vi "Add Rows.vi"(8 "error in (no error)":errorcluster, 10 "Cells":T2(array[cluster]), 11 "DataGridView in":refnum<class "DataGridView.lvclass">) -> (0 "error out":errorcluster, 3 "DataGridView out":refnum<class "DataGridView.lvclass">)   [LabVIEW 2013, in "DataGrid.lvlib" / "DataGridView.lvclass"]
doc: "This method allows you to add any rows of any time, regardless of the data column setup."
uses:
  DataGridView.lvclass
  GridColumn/ColumnType.ctl
  DataGridView.lvclass/DataGridView.ctl
  System.Windows.Forms
  DataTable/DataTable.lvclass
  GridColumn/GridColumn.lvclass
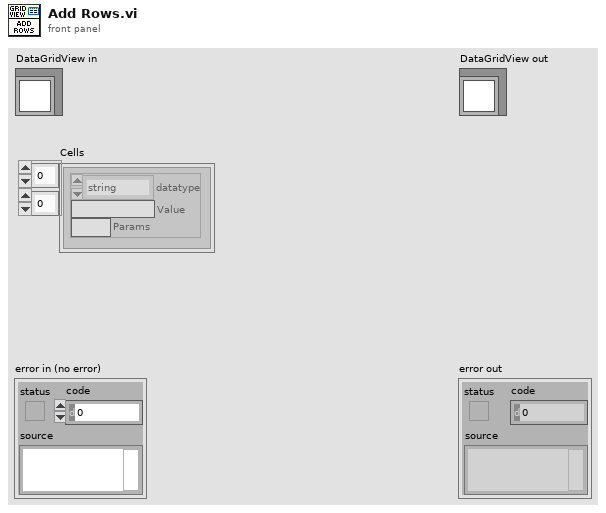
[diagram p1: front panel]
types:
  T1 = typedef "DataGrid.lvlib/GridColumn.lvclass/ColumnType.ctl" = enum16{"string", "image", "check", "numeric", "timestamp", "button", "combo", "link"}
  T2 = cluster{"datatype":T1, "Value":string, "Params":string}[][]
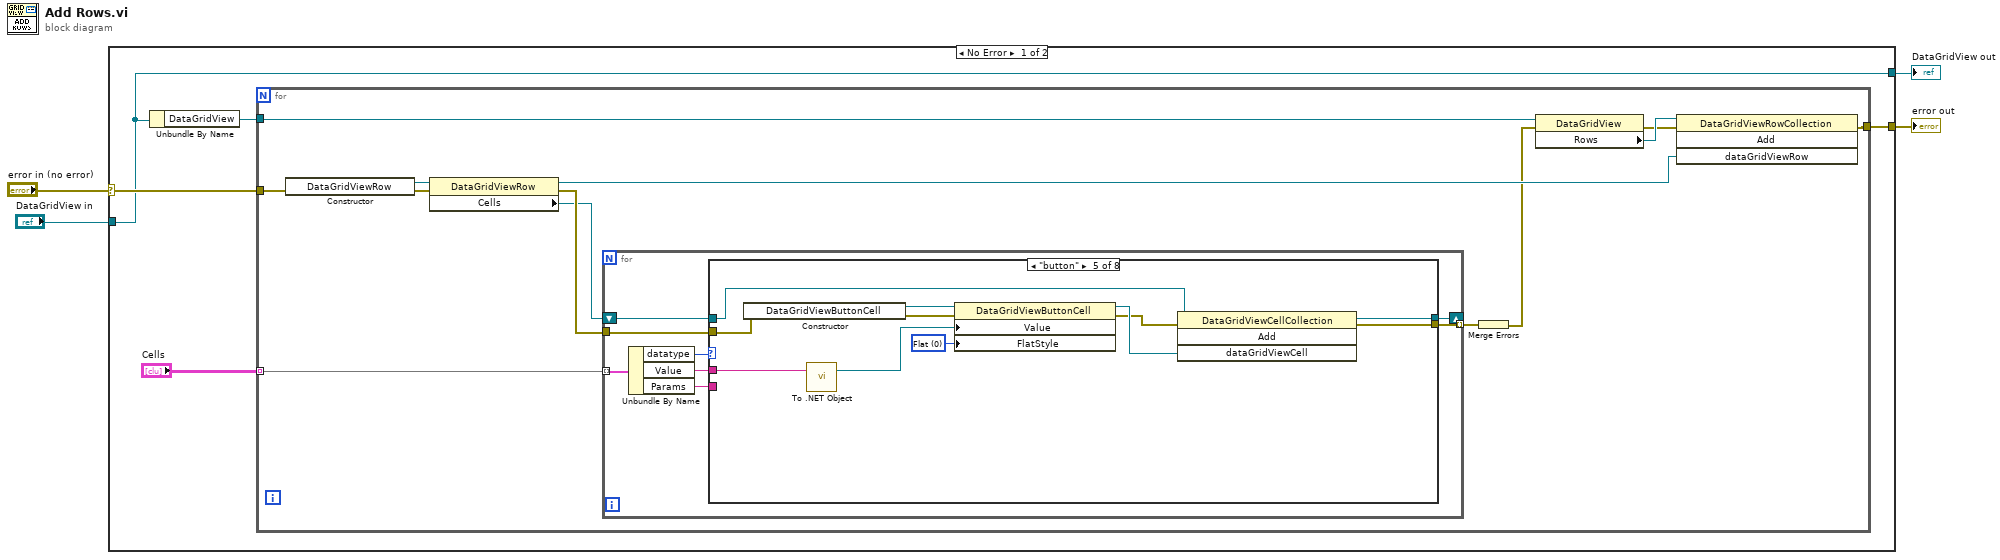
[diagram p0: block diagram]
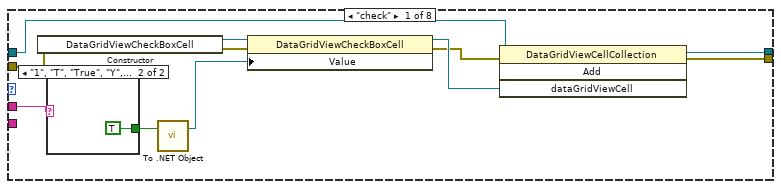
[diagram p2: hidden frame]
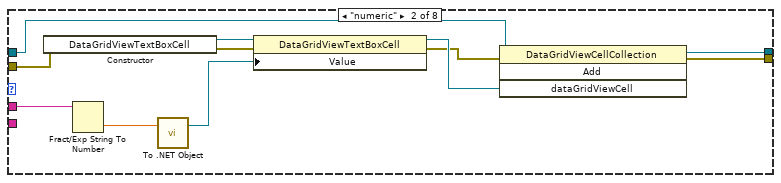
[diagram p4: hidden frame]
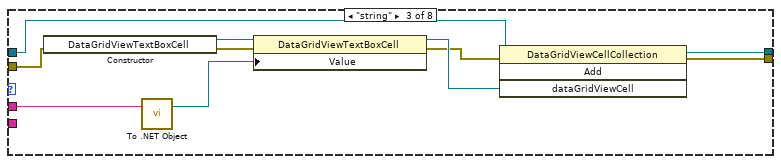
[diagram p5: hidden frame]
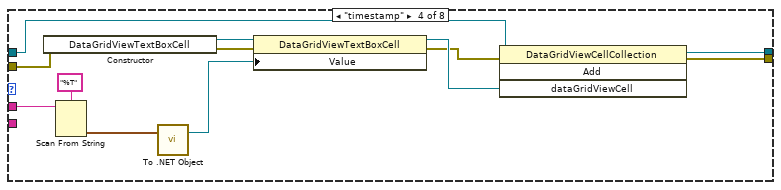
[diagram p6: hidden frame]
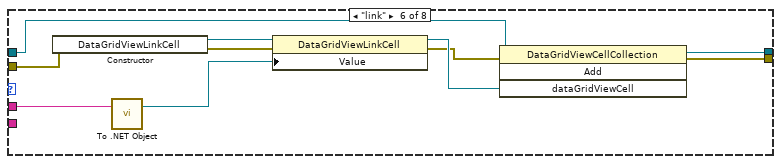
[diagram p7: hidden frame]
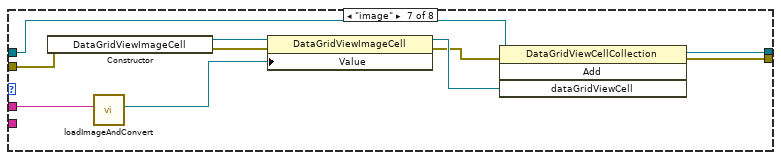
[diagram p8: hidden frame]
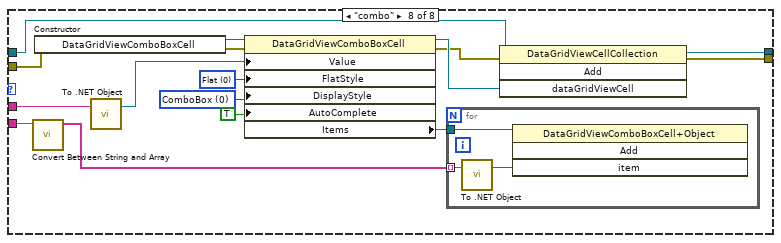
[diagram p9: hidden frame]
diagram:
  n1 = case shown="No Error" "error in (no error)" {
    selector: "error in (no error)" -> [w7 w127]
    tunnel: [w9 w127] -> w3
    tunnel: [w5 w126] -> w1
    tunnel: "DataGridView in" -> [w5 w126]
    frame No Error {
      n2 = Unbundle By Name(w5) -> ("DataGridView"=w8:refnum<k24>)
      n3 = for {
        tunnel: [w22] -> w9
        tunnel: w8 -> [w21]
        tunnel: w7 -> [w17]
        tunnel: "Cells" -> [w10] mode=indexing
        n4 = constructor class="DataGridViewRow"(error in=w17) -> (reference out=w15:refnum<k24>, error out=w16:errorcluster)  [unwired: 2 in, 1 out]
        n5 = property class="DataGridViewRow"(reference=w15, error in=w16) -> (reference out=w14:refnum<k24>, error out=w12:errorcluster, "Cells"=w11:refnum<k24>)
        n6 = for {
          tunnel: w10 -> [w30] mode=indexing
          shift-right: [w26] -> _
          shift-left: w11 -> [w25]
          tunnel: w12 -> [w24]
          tunnel: [w23] -> w19 mode=indexing
          n7 = Unbundle By Name(w30) -> ("datatype"=w29:T1, "Value"=w28:string, "Params"=w27:string)
          n8 = case shown="\"button\"" w29 {
            tunnel: w28 -> [w40 w47 w57 w68 w79 w90 w101 w109]
            tunnel: w27 -> [_ _ _ _ _ _ _ w116]
            tunnel: [w37 w51 w61 w73 w84 w94 w104 w120] -> w26
            tunnel: w25 -> [w35 w49 w59 w71 w82 w92 w102 w118]
            tunnel: w24 -> [w33 w43 w56 w66 w76 w89 w99 w111]
            tunnel: [w31 w45 w54 w65 w77 w87 w98 w113] -> w23
            frame "check" {
              n9 = constructor class="DataGridViewCheckBoxCell"(error in=w33) -> (reference out=w38:refnum<k24>, error out=w39:errorcluster)  [unwired: 2 in, 1 out]
              n10 = case shown="\"1\", \"T\", \"True\", \"Y\", \"Yes\"" w40 {
                tunnel: [_ TRUE] -> w41
                frame Default {
                }
                frame "1", "T", "True", "Y", "Yes" {
                }
              }
              n11 = call <vilib>:"To .NET Object.vi"("anything"=w41) -> (".NET object"=w34:refnum<k24>)  [unwired: 1 in, 1 out]
              n12 = property class="DataGridViewCheckBoxCell"(reference=w38, error in=w39, "Value"=w34) -> (reference out=w36:refnum<k24>, error out=w32:errorcluster)
              n13 = invoke class="DataGridViewCellCollection" method="Add"(reference=w35, error in=w32, "dataGridViewCell"=w36) -> (reference out=w37:refnum<k24>, error out=w31:errorcluster)  [unwired: 1 in, 2 out]
            }
            frame "numeric" {
              n14 = constructor class="DataGridViewTextBoxCell"(error in=w43) -> (reference out=w52:refnum<k24>, error out=w53:errorcluster)  [unwired: 2 in, 1 out]
              n15 = Fract/Exp String To Number(string=w47) -> (number=w46:dbl)  [unwired: 3 in, 1 out]
              n16 = call <vilib>:"To .NET Object.vi"("anything"=w46) -> (".NET object"=w48:refnum<k24>)  [unwired: 1 in, 1 out]
              n17 = property class="DataGridViewTextBoxCell"(reference=w52, error in=w53, "Value"=w48) -> (reference out=w50:refnum<k24>, error out=w44:errorcluster)
              n18 = invoke class="DataGridViewCellCollection" method="Add"(reference=w49, error in=w44, "dataGridViewCell"=w50) -> (reference out=w51:refnum<k24>, error out=w45:errorcluster)  [unwired: 1 in, 2 out]
            }
            frame "string" {
              n19 = constructor class="DataGridViewTextBoxCell"(error in=w56) -> (reference out=w62:refnum<k24>, error out=w63:errorcluster)  [unwired: 2 in, 1 out]
              n20 = call <vilib>:"To .NET Object.vi"("anything"=w57) -> (".NET object"=w58:refnum<k24>)  [unwired: 1 in, 1 out]
              n21 = property class="DataGridViewTextBoxCell"(reference=w62, error in=w63, "Value"=w58) -> (reference out=w60:refnum<k24>, error out=w55:errorcluster)
              n22 = invoke class="DataGridViewCellCollection" method="Add"(reference=w59, error in=w55, "dataGridViewCell"=w60) -> (reference out=w61:refnum<k24>, error out=w54:errorcluster)  [unwired: 1 in, 2 out]
            }
            frame "timestamp" {
              n23 = constructor class="DataGridViewTextBoxCell"(error in=w66) -> (reference out=w74:refnum<k24>, error out=w75:errorcluster)  [unwired: 2 in, 1 out]
              n24 = Scan From String(format string="%T", input string=w68) -> (output 1=w67:timestamp)  [unwired: 3 in, 3 out]
              n25 = call <vilib>:"To .NET Object.vi"("anything"=w67) -> (".NET object"=w70:refnum<k24>)  [unwired: 1 in, 1 out]
              n26 = property class="DataGridViewTextBoxCell"(reference=w74, error in=w75, "Value"=w70) -> (reference out=w72:refnum<k24>, error out=w64:errorcluster)
              n27 = invoke class="DataGridViewCellCollection" method="Add"(reference=w71, error in=w64, "dataGridViewCell"=w72) -> (reference out=w73:refnum<k24>, error out=w65:errorcluster)  [unwired: 1 in, 2 out]
            }
            frame "button" {
              w80 = 0 items=["Flat", "Popup", "Standard", "System"] ("FlatStyle")
              n28 = constructor class="DataGridViewButtonCell"(error in=w76) -> (reference out=w85:refnum<k24>, error out=w86:errorcluster)  [unwired: 2 in, 1 out]
              n29 = call <vilib>:"To .NET Object.vi"("anything"=w79) -> (".NET object"=w81:refnum<k24>)  [unwired: 1 in, 1 out]
              n30 = property class="DataGridViewButtonCell"(reference=w85, error in=w86, "Value"=w81, "FlatStyle"=w80) -> (reference out=w83:refnum<k24>, error out=w78:errorcluster)
              n31 = invoke class="DataGridViewCellCollection" method="Add"(reference=w82, error in=w78, "dataGridViewCell"=w83) -> (reference out=w84:refnum<k24>, error out=w77:errorcluster)  [unwired: 1 in, 2 out]
            }
            frame "link" {
              n32 = constructor class="DataGridViewLinkCell"(error in=w89) -> (reference out=w95:refnum<k24>, error out=w96:errorcluster)  [unwired: 2 in, 1 out]
              n33 = call <vilib>:"To .NET Object.vi"("anything"=w90) -> (".NET object"=w91:refnum<k24>)  [unwired: 1 in, 1 out]
              n34 = property class="DataGridViewLinkCell"(reference=w95, error in=w96, "Value"=w91) -> (reference out=w93:refnum<k24>, error out=w88:errorcluster)
              n35 = invoke class="DataGridViewCellCollection" method="Add"(reference=w92, error in=w88, "dataGridViewCell"=w93) -> (reference out=w94:refnum<k24>, error out=w87:errorcluster)  [unwired: 1 in, 2 out]
            }
            frame "image" {
              n36 = constructor class="DataGridViewImageCell"(error in=w99) -> (reference out=w105:refnum<k24>, error out=w106:errorcluster)  [unwired: 2 in, 1 out]
              n37 = call "loadImageAndConvert.vi"("name or relative path"=w101) -> (".NET object"=w100:refnum<k24>)  [unwired: 9 in, 1 out]
              n38 = property class="DataGridViewImageCell"(reference=w105, error in=w106, "Value"=w100) -> (reference out=w103:refnum<k24>, error out=w97:errorcluster)
              n39 = invoke class="DataGridViewCellCollection" method="Add"(reference=w102, error in=w97, "dataGridViewCell"=w103) -> (reference out=w104:refnum<k24>, error out=w98:errorcluster)  [unwired: 1 in, 2 out]
            }
            frame "combo" {
              w114 = 0 items=["ComboBox", "DropDownButton", "Nothing"] ("DisplayStyle")
              w115 = 0 items=["Flat", "Popup", "Standard", "System"] ("FlatStyle")
              n40 = call "Convert Between String and Array.vi"("String"=w116) -> ("String Array"=w108:string[])  [unwired: 9 in, 1 out]
              n41 = constructor class="DataGridViewComboBoxCell"(error in=w111) -> (reference out=w121:refnum<k24>, error out=w122:errorcluster)  [unwired: 2 in, 1 out]
              n42 = call <vilib>:"To .NET Object.vi"("anything"=w109) -> (".NET object"=w117:refnum<k24>)  [unwired: 1 in, 1 out]
              n43 = property class="DataGridViewComboBoxCell"(reference=w121, error in=w122, "Value"=w117, "FlatStyle"=w115, "DisplayStyle"=w114, "AutoComplete"=TRUE) -> (reference out=w119:refnum<k24>, error out=w112:errorcluster, "Items"=w107:refnum<k24>)
              n44 = for {
                tunnel: w107 -> [w125]
                tunnel: w108 -> [w123] mode=indexing
                n45 = call <vilib>:"To .NET Object.vi"("anything"=w123) -> (".NET object"=w124:refnum<k24>)  [unwired: 1 in, 1 out]
                n46 = invoke class="DataGridViewComboBoxCell+Object" method="Add"(reference=w125, "item"=w124) -> ()  [unwired: 2 in, 4 out]
              }
              n47 = invoke class="DataGridViewCellCollection" method="Add"(reference=w118, error in=w112, "dataGridViewCell"=w119) -> (reference out=w120:refnum<k24>, error out=w113:errorcluster)  [unwired: 1 in, 2 out]
            }
          }
        }
        n48 = Merge Errors(w19) -> (w13:errorcluster)
        n49 = property class="DataGridView"(reference=w21, error in=w13) -> (error out=w18:errorcluster, "Rows"=w20:refnum<k24>)  [unwired: 1 out]
        n50 = invoke class="DataGridViewRowCollection" method="Add"(reference=w20, error in=w18, "dataGridViewRow"=w14) -> (error out=w22:errorcluster)  [unwired: 1 in, 3 out]
      }
    }
    frame Error {
    }
  }
  "error out" <- w3
  "DataGridView out" <- w1
